vi "Simple SFTP File Upload.vi"() -> ()   [LabVIEW 2018]
doc: "Uploads, or sends, a relatively small local file to a remote SFTP server. This is similar to the SFTP command line utility when transferring, or copying, a local file to a remote destination. If performance is poor or memory is limited on the local machine, then it could be because the file is relatively large and this implementation is not very efficient for relatively large files."
uses:
  Toolkit/Type Definitions/Permissions.ctl
  Toolkit/Type Definitions/Modes.ctl
  Toolkit/SFTP File/Type Definitions/Open Options.ctl
  Toolkit/Session/Support/Create from SSH.vi
  Toolkit/Session/Support/Password Authentication.vi
  Toolkit/SFTP/Support/Create from Session.vi
  Toolkit/SFTP File/Support/Open from SFTP.vi
  Toolkit/SFTP File/Support/Close to SFTP.vi
  Toolkit/SFTP/Support/Destroy to Session.vi
  Toolkit/Session/Support/Destroy to SSH.vi
  Toolkit/SSH/SSH.lvclass
  Toolkit/Session/Session.lvclass
  Toolkit/Toolkit.lvlib
  Toolkit/SFTP/SFTP.lvclass
  Toolkit/SFTP File/SFTP File.lvclass
panel:
  in  "Remote File":string
  in  "Local File":path
  in  "Remote SFTP Server":string
  in  "Password":string
  in  "Username":string
  # "Overview: Demonstrates transferring, or uploading, a local file to a remote SFTP server, similar to the SFTP command line utility\nInstructions:\n1. Enter the IP address or host name of the remote SFTP server. This can be a CompactRIO (cRIO) running the National Instruments Linux Real-Time (NI Linux RT) operating system with the Enable Secure Shell Server (sshd) checkbox checked. \n2. Enter a username. If using a cRIO with a default configuration, then the username is \"admin\".\n3. Enter a password for the username. If using a cRIO with a default configuration, then the password is blank (empty).\n4. Select a file on the local computer to transfer/upload to the remote SFTP server.\n5. Enter a path and/or filename for the uploaded file on the remote SFTP server. Typically, this is a POSIX/UNIX file path with a backslash, \"/\", use to separate directories and the default directory is the remote user's home directory, i.e. \"/home/admin\" on a default configured cRIO.\n6. Run this VI."
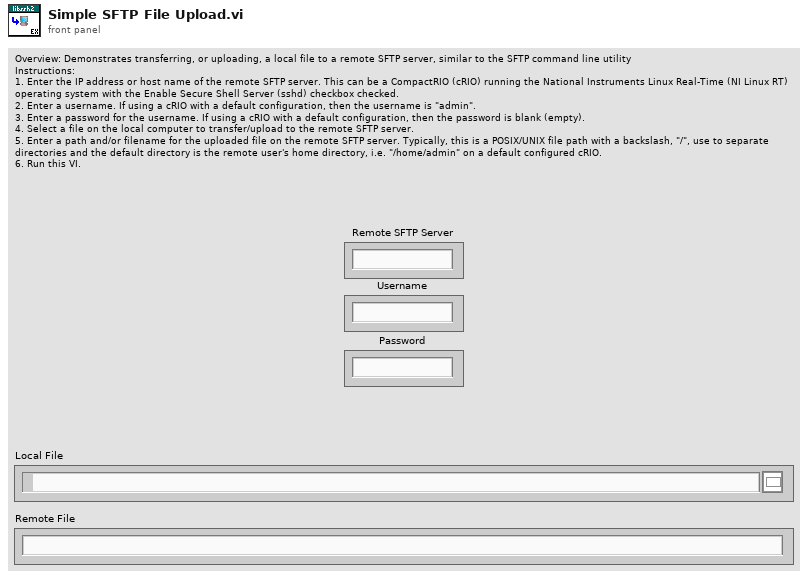
[diagram p1: front panel]
types:
  T1 = typedef "Toolkit.lvlib/SFTP File.lvclass/Open Options.ctl" = cluster{"Read":bool, "Write":bool, "Append":bool, "Create":bool, "Truncate":bool, "Exclude":bool}
  T2 = enum16{"open", "replace", "create", "open or create", "replace or create", "replace or create with confirmation"}
  T3 = typedef "Toolkit.lvlib/Permissions.ctl" = cluster{"Owner":T4, "Group":T4, "Others":T4}
  T4 = typedef "Toolkit.lvlib/Modes.ctl" = cluster{"Read":bool, "Write":bool, "Execute":bool}
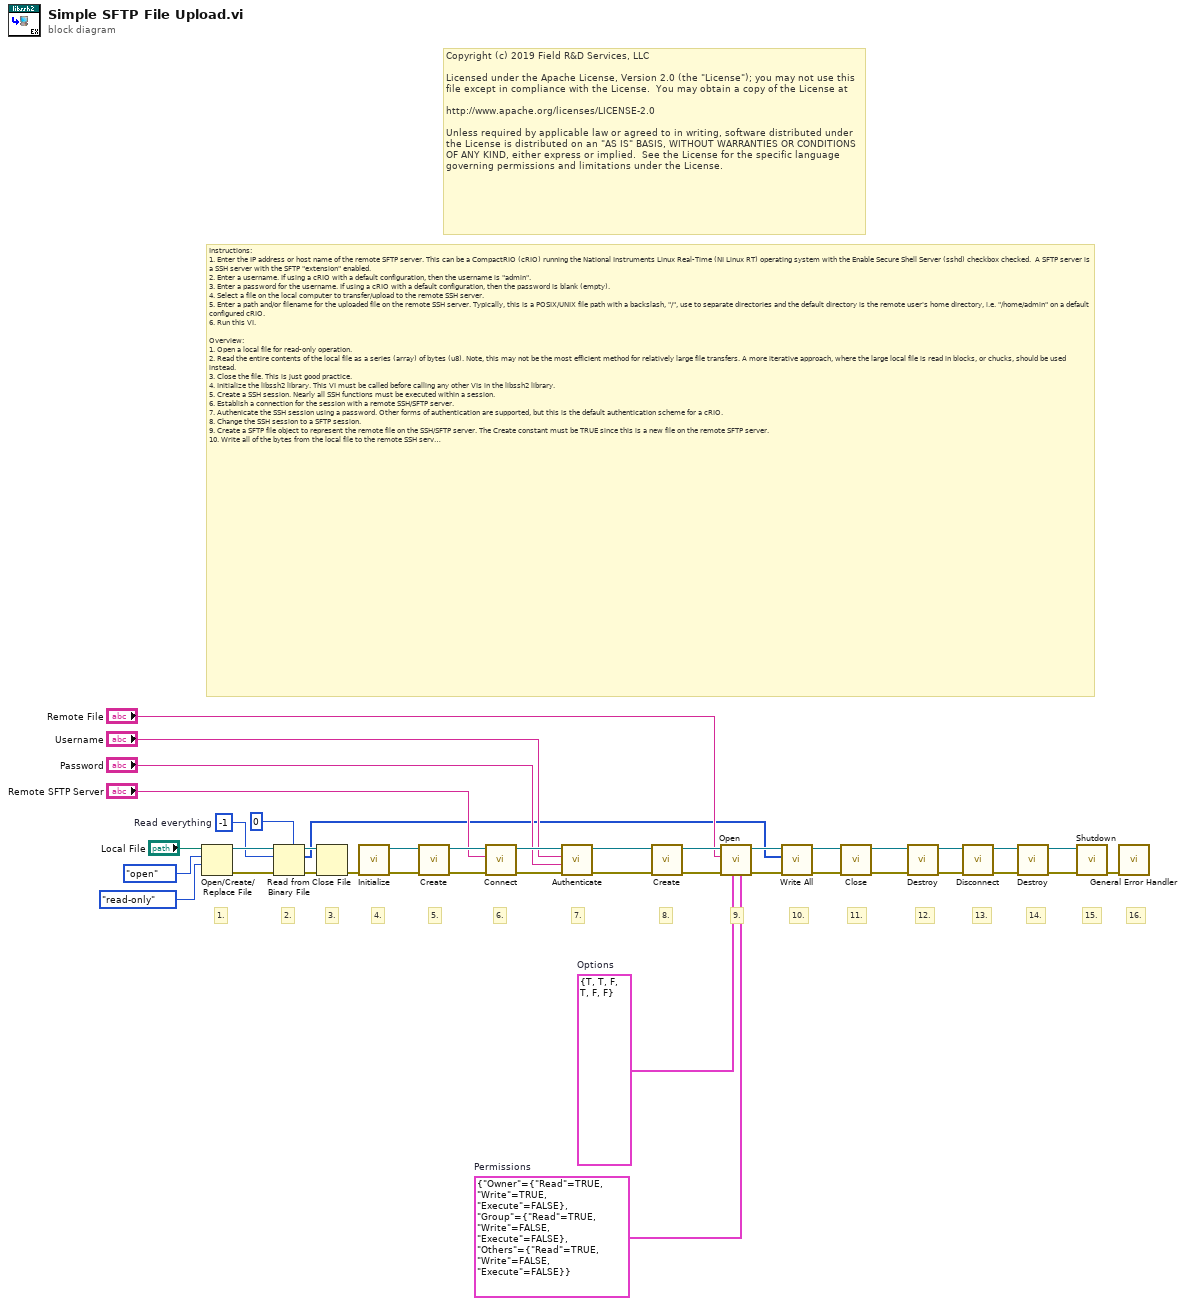
[diagram p0: block diagram]
diagram:
  w10 = T1 {"Read"=TRUE, "Write"=TRUE, "Append"=FALSE, "Create"=TRUE, "Truncate"=FALSE, "Exclude"=FALSE}  # Options
  w30 = -1  # Read everything
  w11 = T3 {"Owner"={"Read"=TRUE, "Write"=TRUE, "Execute"=FALSE}, "Group"={"Read"=TRUE, "Write"=FALSE, "Execute"=FALSE}, "Others"={"Read"=TRUE, "Write"=FALSE, "Execute"=FALSE}}  # Permissions
  # "Copyright (c) 2019 Field R&D Services, LLC\n\nLicensed under the Apache License, Version 2.0 (the \"License\"); you may not use this file except in compliance with the License.  You may obtain a copy of the License at\n\nhttp://www.apache.org/licenses/LICENSE-2.0\n\nUnless required by applicable law or agreed to in writing, software distributed under the License is distributed on an \"AS IS\" BASIS, WITHOUT WARRANTIES OR CONDITIONS OF ANY KIND, either express or implied.  See the License for the specific language governing permissions and limitations under the License."
  # "16."
  # "15."
  # "14."
  # "13."
  # "12."
  # "11."
  # "10."
  # "9."
  # "8."
  # "7."
  # "6."
  # "5."
  # "4."
  # "3."
  # "2."
  # "1."
  # "Instructions:\n1. Enter the IP address or host name of the remote SFTP server. This can be a CompactRIO (cRIO) running the National Instruments Linux Real-Time (NI Linux RT) operating system with the Enable Secure Shell Server (sshd) checkbox checked.  A SFTP server is a SSH server with the SFTP \"extension\" enabled.\n2. Enter a username. If using a cRIO with a default configuration, then the username is \"admin\".\n3. Enter a password for the username. If using a cRIO with a default configuration, then the password is blank (empty).\n4. Select a file on the local computer to transfer/upload to the remote SSH server.\n5. Enter a path and/or filename for the uploaded file on the remote SSH server. Typically, this is a POSIX/UNIX file path with a backslash, \"/\", use to separate directories and the default directory is the remote user's home directory, i.e. \"/home/admin\" on a default configured cRIO.\n6. Run this VI.\n\nOverview:\n1. Open a local file for read-only operation.\n2. Read the entire contents of the local file as a series (array) of bytes (u8). Note, this may not be the most efficient method for relatively large file transfers. A more iterative approach, where the large local file is read in blocks, or chucks, should be used instead.\n3. Close the file. This is just good practice.\n4. Initialize the libssh2 library. This VI must be called before calling any other VIs in the libssh2 library.\n5. Create a SSH session. Nearly all SSH functions must be executed within a session.\n6. Establish a connection for the session with a remote SSH/SFTP server.\n7. Authenicate the SSH session using a password. Other forms of authentication are supported, but this is the default authentication scheme for a cRIO. \n8. Change the SSH session to a SFTP session.\n9. Create a SFTP file object to represent the remote file on the SSH/SFTP server. The Create constant must be TRUE since this is a new file on the remote SFTP server.\n10. Write all of the bytes from the local file to the remote SSH server at the destination specified. Note, this will silently overwrite any existing file on the remote SSH server with the same path and file name.\n11. Close the SFTP file on the remote SSH/SFTP server. Any object that is initialized, opened, or created must be subsequently destroyed, closed, or shutdown to avoid memory leaks, undefined behavior, or crashes.\n12. Change the SFTP session back into a SSH session.\n13. Disconnect from the remote SSH server.\n14. Destroy the session to free resources within the libssh2 library.\n15. Shutdown the libssh2 library. This VI must be last VI called for the libssh2 library. No other libssh2 VIs should be called once this VI is executed.\n16. Provide some error handling and reporting. Libssh2 errors will be in the -8100 range."
  n1 = Open/Create/Replace File(file path (use dialog)="Local File", operation (0:open)=T2."open", access (0:read/write)=enum16{"read/write", "read-only", "write-only"}."read-only") -> (refnum out=w31:refnum<file>, error out=w28:errorcluster)  [unwired: 3 in, 1 out]
  n2 = Read from Binary File(5:u8 0, 8:w28, 10:w30, 11:w31) -> (0:w26:errorcluster, 2:w1:u8[], 3:w27:refnum<file>)  [unwired: 2 in, 1 out]
  n3 = Close File(refnum=w27, error in=w26) -> (error out=w25:errorcluster)  [unwired: 1 out]
  n4 = call "Initialize.vi"("Error In"=w25) -> ("Error Out"=w39:errorcluster, "SSH"=w40:refnum<class "SSH.lvclass">)  [unwired: 9 in]
  n5 = call-poly "Create.vi"("Error In"=w39, "SSH"=w40) -> ("Error Out"=w37:errorcluster, "Sesssion"=w38:refnum<class "Session.lvclass">)  [unwired: 8 in]
  n6 = call "Connect.vi"("Error In"=w37, "Address"="Remote SFTP Server", "Session In"=w38) -> ("Error Out"=w35:errorcluster, "Sesssion Out"=w36:refnum<class "Session.lvclass">)  [unwired: 7 in]
  n7 = call-poly "Authenticate.vi"("Error In"=w35, "Password"="Password", "Username"="Username", "Session In"=w36) -> ("Error Out"=w15:errorcluster, "Sesssion Out"=w16:refnum<class "Session.lvclass">)  [unwired: 6 in]
  n8 = call-poly "Create.vi"("Error In"=w15, "Session"=w16) -> ("Error Out"=w13:errorcluster, "SFTP"=w14:refnum<class "SFTP.lvclass">)  [unwired: 8 in]
  n9 = call-poly "Open.vi"("Permissions"=w11, "Options"=w10, "Error In"=w13, "Remote Path"="Remote File", "SFTP"=w14) -> ("Error Out"=w8:errorcluster, "SFTP File"=w9:refnum<class "SFTP File.lvclass">)  [unwired: 5 in]
  n10 = call "Write All.vi"("Error In"=w8, "Data"=w1, "SFTP File In"=w9) -> ("Error Out"=w6:errorcluster, "SFTP File Out"=w7:refnum<class "SFTP File.lvclass">)  [unwired: 6 in, 1 out]
  n11 = call-poly "Close.vi"("Error In"=w6, "SFTP File"=w7) -> ("Error Out"=w4:errorcluster, "SFTP"=w5:refnum<class "SFTP.lvclass">)  [unwired: 7 in, 1 out]
  n12 = call-poly "Destroy.vi"("Error In"=w4, "SFTP"=w5) -> ("Error Out"=w2:errorcluster, "Session"=w3:refnum<class "Session.lvclass">)  [unwired: 8 in]
  n13 = call "Disconnect.vi"("Error In"=w2, "Session In"=w3) -> ("Error Out"=w23:errorcluster, "Sesssion Out"=w24:refnum<class "Session.lvclass">)  [unwired: 8 in]
  n14 = call-poly "Destroy.vi"("Error In"=w23, "Session"=w24) -> ("Error Out"=w21:errorcluster, "SSH"=w22:refnum<class "SSH.lvclass">)  [unwired: 8 in]
  n15 = call "Shutdown.vi"("Error In"=w21, "SSH"=w22) -> ("Error Out"=w20:errorcluster)  [unwired: 9 in]
  n16 = call <vilib>:"General Error Handler.vi"("error in (no error)"=w20) -> ()  [unwired: 10 in, 5 out]
